vi "motor_id.vi"() -> ()   [LabVIEW 2014]
uses:
  <vilib>/rvi/FXPMathLib/FxpSinAndCos/subVIs/nifxpmath_SinAndCos_SimConfig.ctl
  <vilib>/rvi/Emulation/niFpgaGetClockAttributes.vi
  <vilib>/rvi/Emulation/niFpgaSctlEmulationGetInTimedLoop.vi
  <vilib>/rvi/Emulation/niFpgaEmulationReportErrorSimple.vi
  <vilib>/rvi/eio/common/nirviEmuTemplateMethod_errors.vi
  <vilib>/rvi/Emulation/niFpgaProcessEmulError.vi
  <vilib>/rvi/Emulation/niFpgaCriticalErrorInLSC.vi
  <vilib>/rvi/interface/RandomDataEmulation/nirviRandomDataMultiElementFPGAFIFO.vi
  <instcachedir>/0/nirviRandomDataMultiElementFPGAFIFO_AD0CFC12EF974623A9C2E4184BC062B2.lvgen/nirviRandomDataMultiElementFPGAFIFO_AD0CFC12EF974623A9C2E4184BC062B2_006.vi
  <vilib>/rvi/interface/RandomDataEmulation/niFpgaRandomDataHandleErrors.vi
  <vilib>/rvi/FXPMathLib/FxpSinAndCos/simVIs/DllFxpSinAndCosTemp_sub.vi
  <vilib>/eio/EIONode/EIONode.xnode
  <vilib>/rvi/FXPMathLib/FxpMul/XNode/nifxpmath_Multiplier.xnode
  <vilib>/rvi/DataTransferAndStorage/Container/XNode/niFpgaContainer.xnode
  <vilib>/rvi/interface/RandomDataEmulation/nirviRandomDataFpgaMultiElementTemplate.vi
  <vilib>/rvi/FXPMathLib/FxpSinAndCos/XNode/nifxpmath_SinAndCos.xnode
  <vilib>/rvi/Analysis/measure/butterworth/XNode/niFpgaButterworthFilter.xnode
  <vilib>/rvi/FXPMathLib/sim/FxpSim.dll
panel:
  in  "Current filter coefficients":i32[](array[numeric])=[-1072788146, 2146529546, 106]
  out "iq":fxp<+/-,21,6>
  out "id":fxp<+/-,21,6>
  out "ib":fxp<+/-,51,21>
  out "ia":fxp<+/-,51,21>
  in  "Current Sensor Coe_b":fxp<+/-,26,11>
  in  "Current Sensor Coe_a":fxp<+/-,26,11>
  out "vib":fxp<+/-,25,10>
  out "via":fxp<+/-,25,10>
  in  "Current Sensor Reset":bool
  in  "Current Filter on/off":bool
  in  "Current Filter reset":bool
  in  "Dp stroke (mm)":fxp<+,22,7>
  out "Vp (mm/s)":fxp<+/-,41,8>
  in  "Coe Ini":bool
  in  "Encoder Reset":bool
  in  "Stop Motor":bool
  out "Encoder Position":i32 format="%#_6f"
  out "rad(NrTheta)":fxp<+/-,33,18> format="%.21g"
  out "Dp (mm)":fxp<+/-,22,7>
  out "omega":fxp<+/-,20,9>
  in  "vq_const":fxp<+/-,20,5>
  in  "vd_const":fxp<+/-,20,5>
  out "va":fxp<+/-,37,7>
  out "vb":fxp<+/-,38,8>
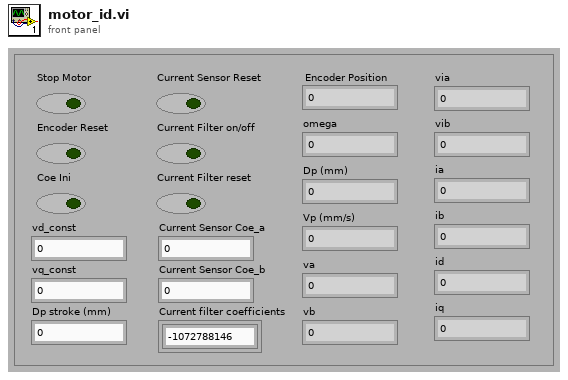
[diagram p1: front panel]
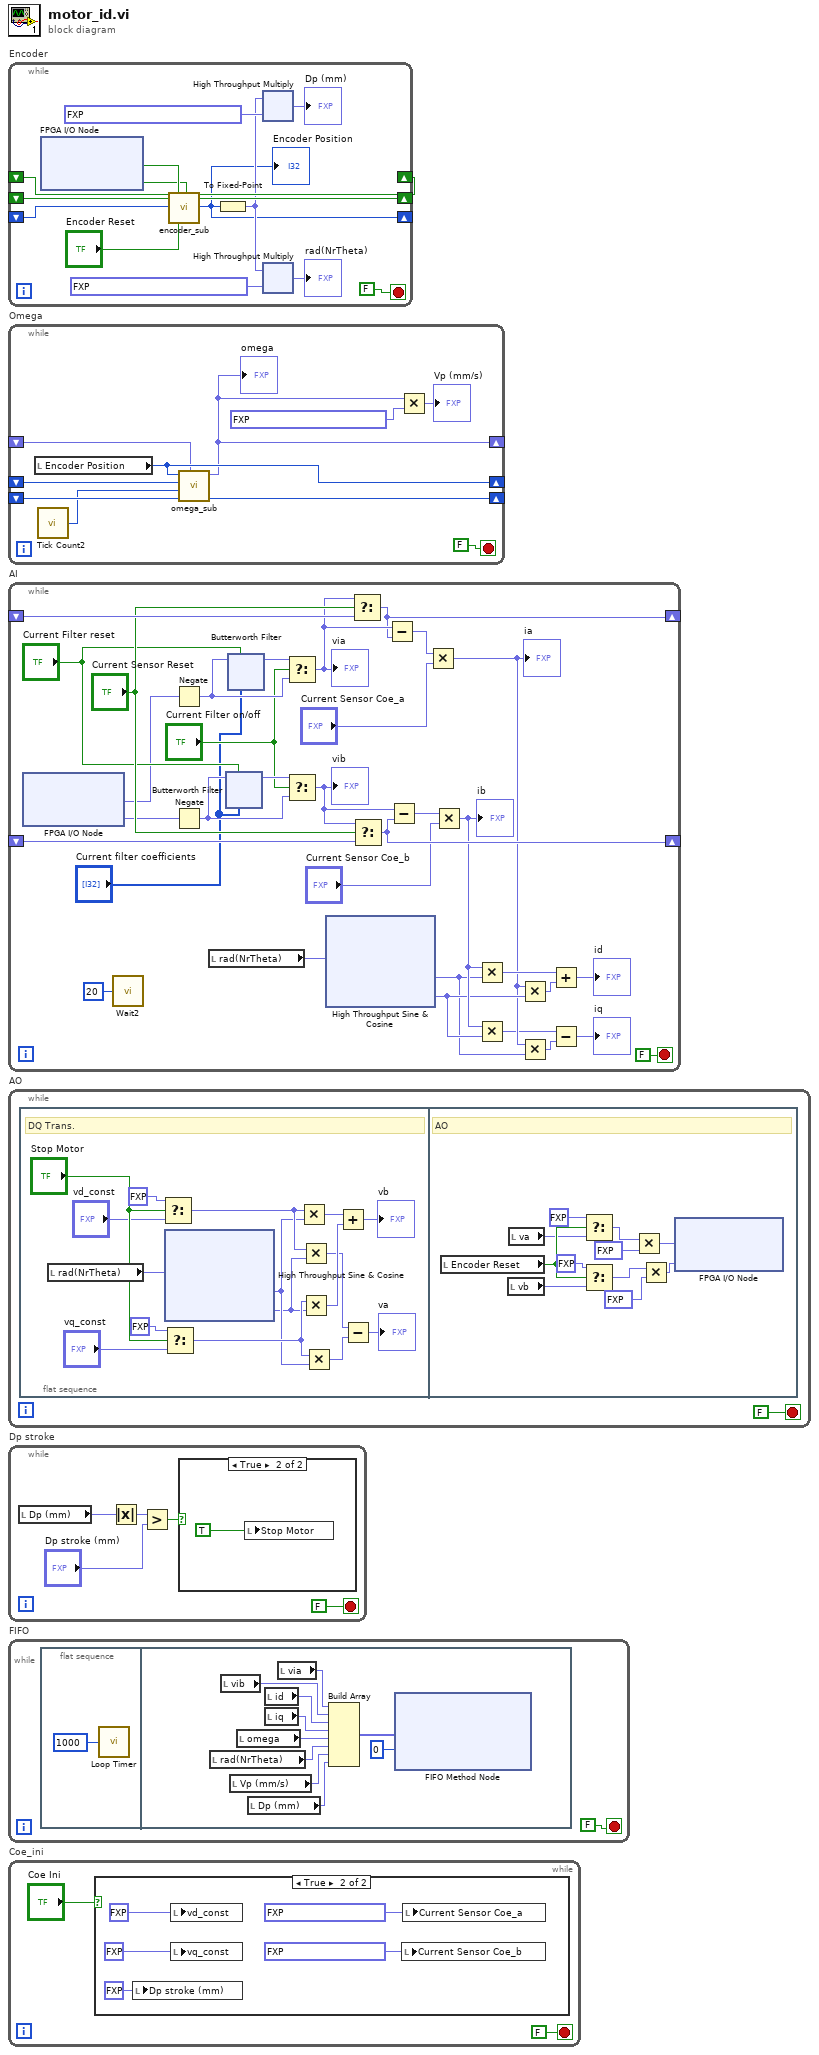
[diagram p0: block diagram]
diagram:
  n1 = while "Encoder" {
    shift-right: [w14] -> _
    shift-left: _ -> [w12]
    shift-right: [w13] -> _
    shift-left: _ -> [w11]
    shift-right: [w4] -> _
    shift-left: _ -> [w10]
    stop <- FALSE stop-if-true
    n2 = xnode "FPGA I/O Node"() -> ("Mod2/DI3"=w2:bool, "Mod2/DI4"=w1:bool)  [unwired: 2 in, 2 out]
    n3 = call "encoder_sub.vi"("A_pre"=w12, "B_pre"=w11, "Encoder Position_pre"=w10, "A input"=w2, "Encoder Position Reset"="Encoder Reset", "B input"=w1) -> ("A"=w14:bool, "B"=w13:bool, "Encoder Position (Counts)"=w4:i32)  [unwired: 19 in]
    "Encoder Position" <- w4
    n4 = To Fixed-Point(number=w4) -> (fixed-point=w7:fxp<+/-,18,18>)  [unwired: 1 in]
    n5 = xnode ("High Throughput Multiply")("x"=w7, "y"=fxp<+/-,15,-9> 0.0006350278854370117) -> ("x*y"=→"Dp (mm)":fxp<+/-,22,7>)
    n6 = xnode ("High Throughput Multiply")("x"=w7, "y"=fxp<+,24,0> 0.02499997615814209) -> ("x*y"=→"rad(NrTheta)":fxp<+/-,33,18>)
  }
  n7 = while "Omega" {
    shift-right: [w25] -> _
    shift-left: _ -> [w24]
    shift-right: [w23] -> _
    shift-left: _ -> [w22]
    shift-right: [w16] -> _
    shift-left: _ -> [w21]
    stop <- FALSE stop-if-true
    n8 = local read "Encoder Position"() -> (w25:i32)
    n9 = call "Tick Count2"() -> ("Tick Count(Ticks)"=w19:u32)
    n10 = call "omega_sub.vi"("omega_pre"=w21, "ticks_m_pre"=w22, "ticks"=w19, "count_pre"=w24, "count"=w25) -> ("ticks_m"=w23:u32, "omega"=w16:fxp<+/-,20,9>)  [unwired: 5 in]
    "omega" <- w16
    n11 = Multiply(x=w16, y=fxp<+,21,-1> 0.4042539596557617) -> (x*y=→"Vp (mm/s)":fxp<+/-,41,8>)
  }
  n12 = while "AI" {
    shift-right: [w46] -> _
    shift-left: _ -> [w51]
    shift-right: [w42] -> _
    shift-left: _ -> [w50]
    stop <- FALSE stop-if-true
    n13 = xnode "FPGA I/O Node"() -> ("Mod5/AI0"=w27:fxp<+/-,20,5>, "Mod5/AI1"=w28:fxp<+/-,20,5>)  [unwired: 2 in, 2 out]
    n14 = call "Wait2"("Count(uSec)"=u32 20) -> ()  [unwired: 1 out]
    n15 = Negate(x=w27) -> (-x=w55:fxp<+/-,21,6>)
    n16 = Negate(x=w28) -> (-x=w53:fxp<+/-,21,6>)
    n17 = local read "rad(NrTheta)"() -> (w57:fxp<+/-,33,18>)
    n18 = xnode "Butterworth Filter"("input data"=w53, "reset"="Current Filter reset", "scaled coefficients"="Current filter coefficients") -> ("output data"=w54:fxp<+/-,25,10>)
    n19 = xnode "Butterworth Filter"("input data"=w55, "reset"="Current Filter reset", "scaled coefficients"="Current filter coefficients") -> ("output data"=w56:fxp<+/-,25,10>)
    n20 = Select(t=w56, s="Current Filter on/off", f=w55) -> (s? t:f=w48:fxp<+/-,25,10>)
    "via" <- w48
    n21 = Select(t=w54, s="Current Filter on/off", f=w53) -> (s? t:f=w43:fxp<+/-,25,10>)
    "vib" <- w43
    n22 = xnode "High Throughput Sine & Cosine"("x (pi)"=w57) -> ("sin(x)"=w33:fxp<+/-,17,2>, "cos(x)"=w37:fxp<+/-,17,2>)
    n23 = Select(t=w48, s="Current Sensor Reset", f=w51) -> (s? t:f=w46:fxp<+/-,25,10>)
    n24 = Select(t=w43, s="Current Sensor Reset", f=w50) -> (s? t:f=w42:fxp<+/-,25,10>)
    n25 = Subtract(x=w48, y=w46) -> (x-y=w45:fxp<+/-,26,11>)
    n26 = Subtract(x=w43, y=w42) -> (x-y=w41:fxp<+/-,26,11>)
    n27 = Multiply(x=w45, y="Current Sensor Coe_a") -> (x*y=w34:fxp<+/-,51,21>)
    "ia" <- w34
    n28 = Multiply(x=w41, y="Current Sensor Coe_b") -> (x*y=w38:fxp<+/-,51,21>)
    "ib" <- w38
    n29 = Multiply(x=w38, y=w33) -> (x*y=w36:fxp<+/-,20,5>)
    n30 = Multiply(x=w38, y=w37) -> (x*y=w32:fxp<+/-,20,5>)
    n31 = Multiply(x=w34, y=w37) -> (x*y=w35:fxp<+/-,20,5>)
    n32 = Multiply(x=w34, y=w33) -> (x*y=w31:fxp<+/-,20,5>)
    n33 = Add(x=w36, y=w35) -> (x+y=→"id":fxp<+/-,21,6>)
    n34 = Subtract(x=w32, y=w31) -> (x-y=→"iq":fxp<+/-,21,6>)
  }
  n35 = while "AO" {
    stop <- FALSE stop-if-true
    n36 = flat-sequence {
      frame #0 {
        # "DQ Trans."
        n37 = local read "rad(NrTheta)"() -> (w121:fxp<+/-,33,18>)
        n38 = Select(t=fxp<+/-,20,5> 0.0, s="Stop Motor", f="vd_const") -> (s? t:f=w118:fxp<+/-,20,5>)
        n39 = xnode "High Throughput Sine & Cosine"("x (pi)"=w121) -> ("sin(x)"=w116:fxp<+/-,17,2>, "cos(x)"=w115:fxp<+/-,17,2>)
        n40 = Select(t=fxp<+/-,20,5> 0.0, s="Stop Motor", f="vq_const") -> (s? t:f=w117:fxp<+/-,20,5>)
        n41 = Multiply(x=w118, y=w116) -> (x*y=w114:fxp<+/-,37,7>)
        n42 = Multiply(x=w118, y=w115) -> (x*y=w112:fxp<+/-,37,7>)
        n43 = Multiply(x=w117, y=w115) -> (x*y=w113:fxp<+/-,37,7>)
        n44 = Multiply(x=w117, y=w116) -> (x*y=w111:fxp<+/-,37,7>)
        n45 = Add(x=w114, y=w113) -> (x+y=→"vb":fxp<+/-,38,8>)
        n46 = Subtract(x=w112, y=w111) -> (x-y=→"va":fxp<+/-,37,7>)
      }
      frame #1 {
        # "AO"
        n47 = local read "Encoder Reset"() -> (w156:bool)
        n48 = local read "vb"() -> (w154:fxp<+/-,38,8>)
        n49 = local read "va"() -> (w155:fxp<+/-,37,7>)
        n50 = Select(t=fxp<+/-,37,7> 5.0, s=w156, f=w155) -> (s? t:f=w158:fxp<+/-,37,7>)
        n51 = Select(t=fxp<+/-,38,8> 0.0, s=w156, f=w154) -> (s? t:f=w161:fxp<+/-,38,8>)
        n52 = Multiply(x=w158, y=fxp<+/-,20,5> -0.5) -> (x*y=w157:fxp<+/-,20,5>)
        n53 = Multiply(x=w161, y=fxp<+/-,20,5> -0.5) -> (x*y=w162:fxp<+/-,20,5>)
        n54 = xnode "FPGA I/O Node"("Mod1/AO0"=w157, "Mod1/AO1"=w162) -> ()  [unwired: 2 in, 2 out]
      }
    }
  }
  n55 = while "Dp stroke" {
    stop <- FALSE stop-if-true
    n56 = local read "Dp (mm)"() -> (w166:fxp<+/-,22,7>)
    n57 = Absolute Value(x=w166) -> (abs(x)=w165:fxp<+,22,7>)
    n58 = Greater?(x=w165, y="Dp stroke (mm)") -> (0:w163:bool)
    n59 = case shown="True" w163 {
      frame False {
      }
      frame True {
        n60 = local write "Stop Motor"(TRUE ("Stop Motor_p")) -> ()
      }
    }
  }
  n61 = while "FIFO" {
    stop <- FALSE stop-if-true
    n62 = flat-sequence {
      frame #0 {
        n63 = call "Loop Timer"("Count(uSec)"=u32 1000 ("Loop Period (usec)")) -> ()  [unwired: 1 out]
      }
      frame #1 {
        n64 = local read "rad(NrTheta)"() -> (w173:fxp<+/-,33,18>)
        n65 = local read "vib"() -> (w177:fxp<+/-,25,10>)
        n66 = local read "Vp (mm/s)"() -> (w172:fxp<+/-,41,8>)
        n67 = local read "omega"() -> (w174:fxp<+/-,20,9>)
        n68 = local read "Dp (mm)"() -> (w171:fxp<+/-,22,7>)
        n69 = local read "id"() -> (w176:fxp<+/-,21,6>)
        n70 = local read "iq"() -> (w175:fxp<+/-,21,6>)
        n71 = local read "via"() -> (w178:fxp<+/-,25,10>)
        n72 = Build Array(w178, w177, w176, w175, w174, w173, w172, w171) -> (w179:fxp<+/-,51,18>[])
        n73 = xnode ("FIFO Method Node")("Element"=w179, "Timeout"=0) -> ()  [unwired: 1 in, 2 out]
      }
    }
  }
  n74 = while "Coe_ini" {
    stop <- FALSE stop-if-true
    n75 = case shown="True" "Coe Ini" {
      frame False {
      }
      frame True {
        n76 = local write "Dp stroke (mm)"(fxp<+,22,7> 5.0 ("Dp stroke (mm)")) -> ()
        n77 = local write "vd_const"(fxp<+/-,20,5> -2.0 ("vd_const")) -> ()
        n78 = local write "vq_const"(fxp<+/-,20,5> 5.0 ("vq_const")) -> ()
        n79 = local write "Current Sensor Coe_b"(fxp<+/-,26,11> 0.579742431640625 ("Current Sensor Coe_b")) -> ()
        n80 = local write "Current Sensor Coe_a"(fxp<+/-,26,11> 0.578155517578125 ("Current Sensor Coe_a")) -> ()
      }
    }
  }
